vi "Reverse Swerve.vi"(8 "error in (no error)":errorcluster, 10 "POSold":dbl, 11 "Joystick Value":dbl) -> (0 "error out":errorcluster, 1 "Reversed":bool, 3 "POSnew":dbl)   [LabVIEW 2023]
uses:
  <vilib>/Analysis/coordinate.llb/Angle Units.ctl
  <vilib>/Analysis/coordinate.llb/Angle Range (Degree).ctl
  <vilib>/Analysis/coordinate.llb/Wrap Angle (scalar).vi
  <vilib>/Analysis/NI_AAL_Angle.lvlib
panel:
  out "min index(es)":i32
  out "Delta":dbl[](array[numeric])
  out "Min value(abs)":dbl
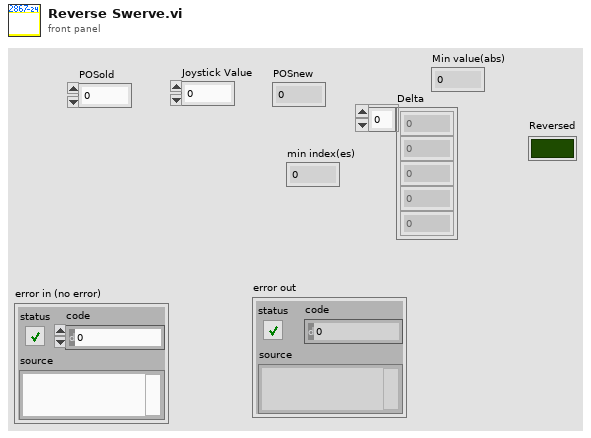
[diagram p1: front panel]
types:
  T1 = typedef "NI_AAL_Angle.lvlib/Angle Range (Degree).ctl" = u16
  T2 = typedef "NI_AAL_Angle.lvlib/Angle Units.ctl" = i32
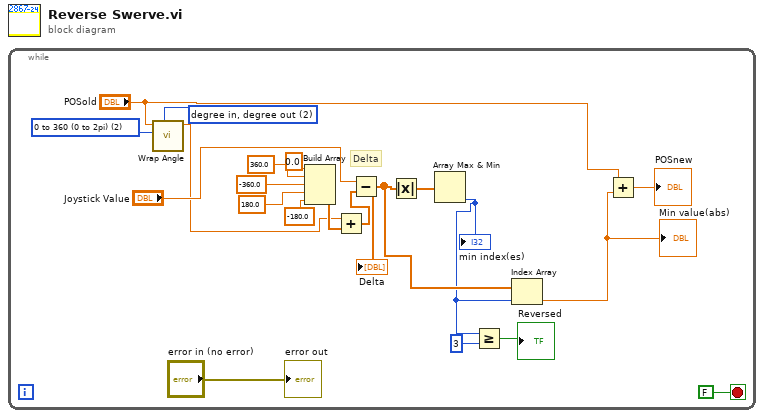
[diagram p0: block diagram]
diagram:
  n1 = while {
    stop <- FALSE stop-if-true
    w6 = T1 2 items=["none", "-180 to 180 (-pi to pi)", "0 to 360 (0 to 2pi)"] ("angle range")
    w7 = T2 2 items=["radian in, radian out", "radian in, degree out", "degree in, degree out", "degree in, radian out"] ("angle units")
    # "Delta"
    n2 = call-poly <vilib>:"Wrap Angle.vi"("angle units"=w7, "angle range"=w6, "angle in"="POSold") -> ("angle out"=w3:dbl)  [unwired: 7 in, 1 out]
    n3 = Build Array(0.0 ("element"), 360.0 ("element"), -360.0 ("element"), 180.0 ("element"), -180.0 ("element")) -> (w4:dbl[])
    n4 = Add(x=w3, y=w4) -> (x+y=w2:dbl[])
    n5 = Subtract(x="Joystick Value", y=w2) -> (x-y=w12:dbl[])
    "Delta" <- w12
    n6 = Absolute Value(x=w12) -> (abs(x)=w13:dbl[])
    n7 = Array Max & Min(array=w13) -> (min index (indices)=w10:i32)  [unwired: 3 out]
    "min index(es)" <- w10
    n8 = Greater Or Equal?(x=w10, y=3) -> (x >= y?=→"Reversed":bool)
    n9 = Index Array(array=w12, index=w10) -> (element=w11:dbl)
    "Min value(abs)" <- w11
    n10 = Add(x="POSold", y=w11) -> (x+y=→"POSnew":dbl)
    "error out" <- "error in (no error)"
  }
